vi "triatge 3_dades.vi"(8 "Cluster - Borderless":T1, 11 "DataIN":string) -> (0 "ShiftReg Right":T2, 3 "Acceleròmetre":cluster{dbl, dbl, dbl}(graph)={-1477.92, 1162.76, -1186.5} caption="Waveform Chart - Dark", 4 "String Out":string)   [LabVIEW 2018]
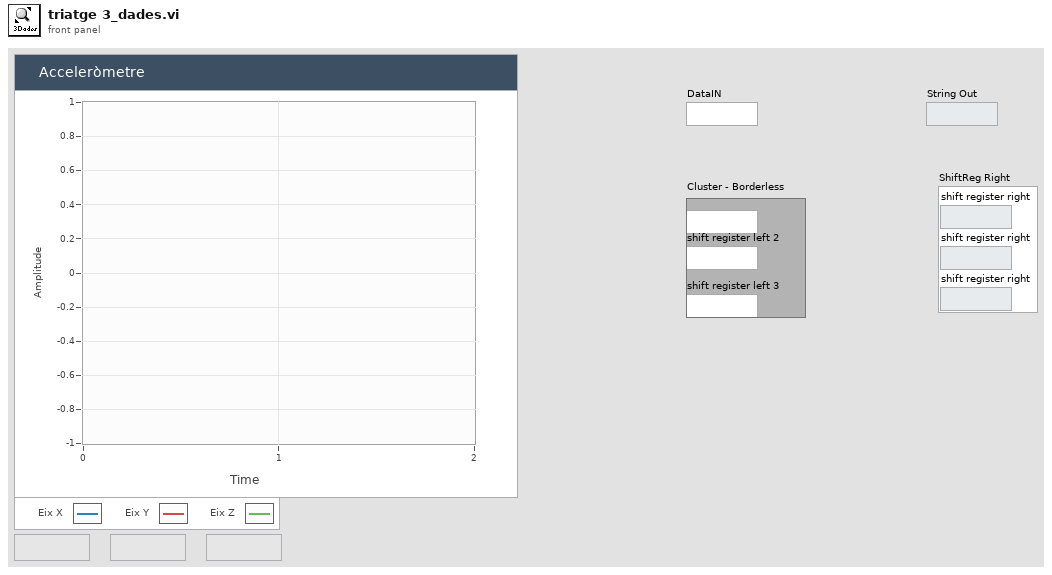
[diagram p1: front panel]
types:
  T1 = cluster{"shift register left":string, "shift register left 2":string, "shift register left 3":string}
  T2 = cluster{"shift register right":string, "shift register right":string, "shift register right":string}
  T3 = cluster{"Data Out":dbl, "Data Out":dbl, "Data Out":dbl}
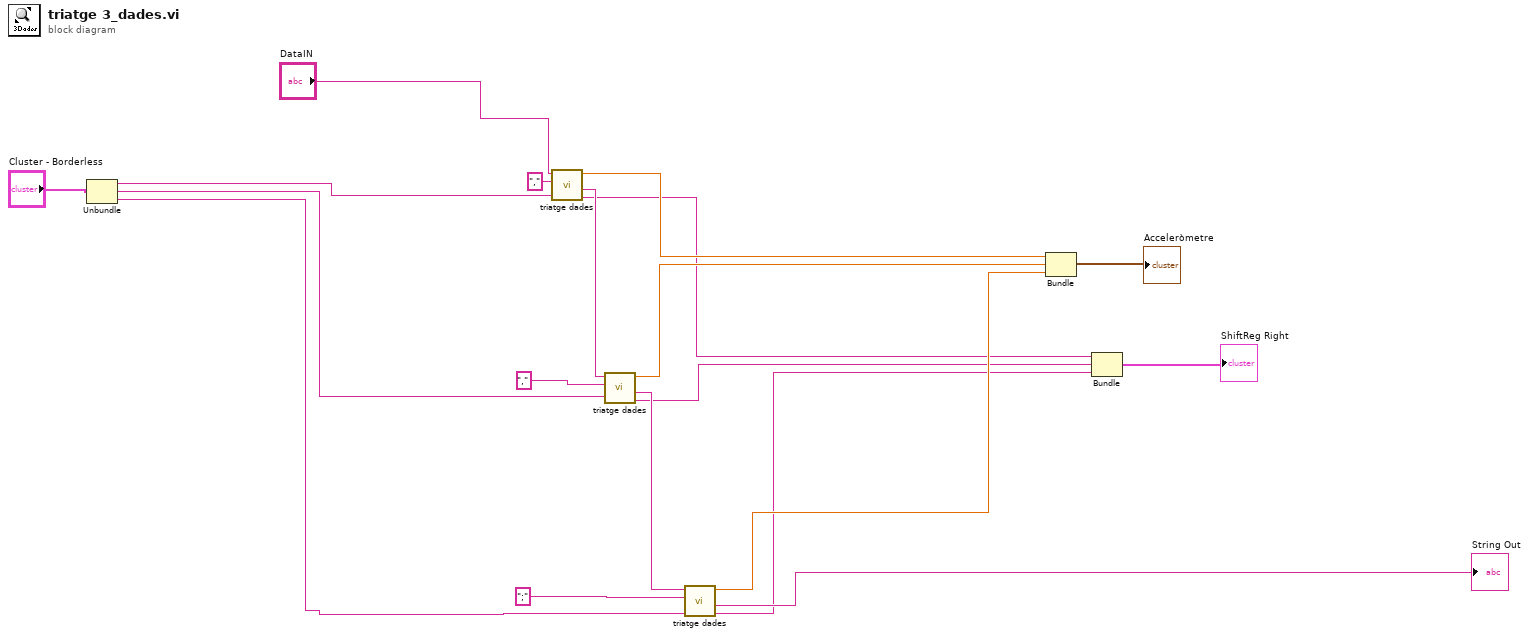
[diagram p0: block diagram]
diagram:
  n1 = Unbundle("Cluster - Borderless") -> ("shift register left"=w4:string, "shift register left 2"=w2:string, "shift register left 3"=w1:string)
  n2 = call "triatge dades.vi"("shift register left"=w4, "dada a buscar"=",", "String in"="DataIN") -> ("shift register right"=w8:string, "String Out"=w16:string, "Data Out"=w18:dbl)  [unwired: 5 in, 1 out]
  n3 = call "triatge dades.vi"("shift register left"=w2, "dada a buscar"=",", "String in"=w16) -> ("shift register right"=w7:string, "String Out"=w14:string, "Data Out"=w13:dbl)  [unwired: 5 in, 1 out]
  n4 = call "triatge dades.vi"("shift register left"=w1, "dada a buscar"=";", "String in"=w14) -> ("shift register right"=w6:string, "String Out"=→"String Out":string, "Data Out"=w12:dbl)  [unwired: 5 in, 1 out]
  n5 = Bundle("Data Out"=w18, "Data Out"=w13, "Data Out"=w12) -> (→"Acceleròmetre":T3)  [unwired: 1 in]
  n6 = Bundle("shift register right"=w8, "shift register right"=w7, "shift register right"=w6) -> (→"ShiftReg Right":T2)  [unwired: 1 in]
